vi "LTESaveDataImg2.vi"(7 "Boolean":bool, 8 "error in":errorcluster, 9 "varName":string, 10 "2-D Array of Complex":cdb[][](array[numeric]), 11 "Path":path=path "C:/Users/Administrator/Desktop") -> (0 "error IO":errorcluster)   [LabVIEW 2015]
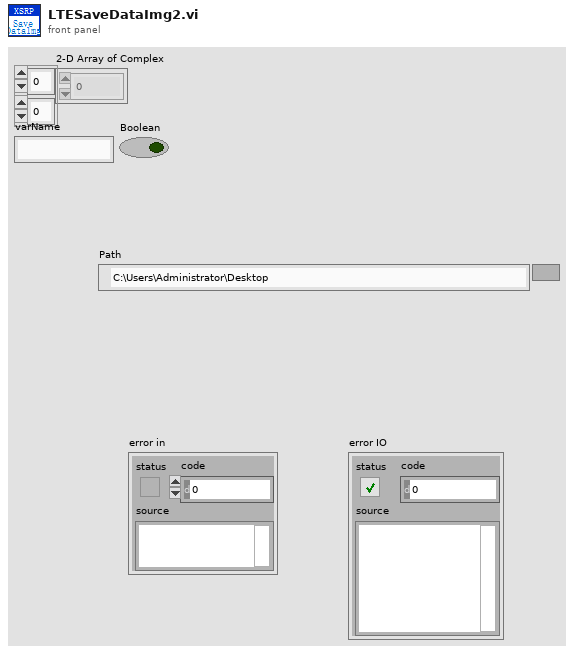
[diagram p1: front panel]
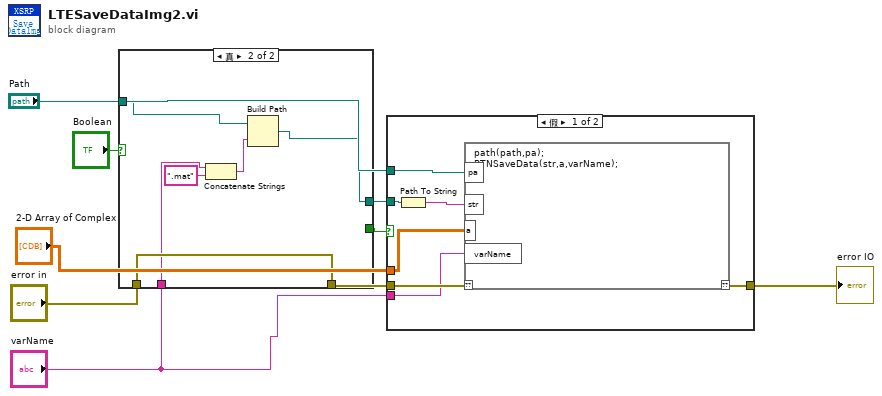
[diagram p0: block diagram]
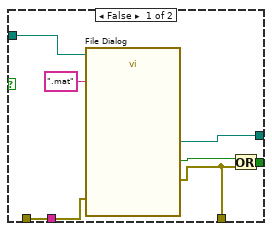
[diagram p2: hidden frame]
diagram:
  n1 = case shown="真" "Boolean" {
    tunnel: [w16 w18] -> w9
    tunnel: [w14 _] -> w8
    tunnel: "Path" -> [w13 w19]
    tunnel: "error in" -> [w12 w22]
    tunnel: [w11 w22] -> w4
    tunnel: "varName" -> [_ w17]
    frame False {
      n2 = call "File Dialog"("start path"=w13, "error in"=w12, "pattern (all files)"=".mat") -> ("selected path"=w16:path, "cancelled"=w10:bool, "error out"=w11:errorcluster)  [unwired: 9 in, 1 out]
      n3 = Or(x=w10, y=w11) -> (x .or. y?=w14:bool)
    }
    frame True {
      n4 = Concatenate Strings(w17, ".mat" ("string")) -> (w20:string)
      n5 = Build Path(base path=w19, name or relative path=w20) -> (appended path=w18:path)
    }
  }
  n6 = case shown="假" w8 {
    tunnel: w9 -> [w29 _]
    tunnel: "Path" -> [w27 _]
    tunnel: w4 -> [w26 w30]
    tunnel: [w25 w30] -> w6
    tunnel: "2-D Array of Complex" -> [w24 _]
    tunnel: "varName" -> [w23 _]
    frame False {
      n7 = Path To String(path=w29) -> (string=w28:string)
      n8 = script code="path(path,pa);\nBTNSaveData(str,a,varName);"("??"=w26, "pa"=w27, "a"=w24, "str"=w28, "varName"=w23) -> ("??"=w25:errorcluster)
    }
    frame True {
    }
  }
  "error IO" <- w6
